vi "Display and Log Custom Device Error (Filtered).vi"(8 "error in (no error)":errorcluster, 9 "Note (empty)":string, 10 "Your code's public name":string) -> ()   [LabVIEW 2015, in "J1939 Addon Engine.lvlib" / "Error Handling API.lvlib"]
uses:
  Error Handling API.lvlib
  <vilib>/NI Veristand/Custom Device Tools/Custom Device Utility Library/NI VeriStand - Print Debug String.vi
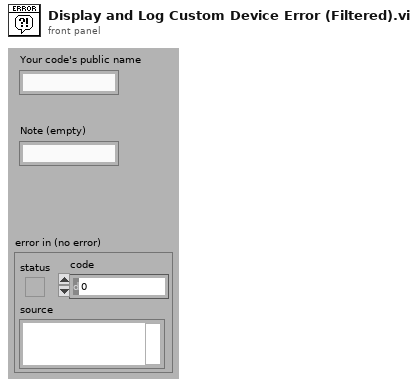
[diagram p1: front panel]
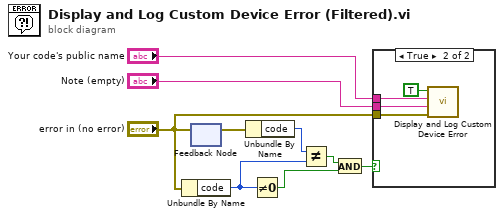
[diagram p0: block diagram]
diagram:
  n1 = Unbundle By Name("error in (no error)") -> ("code"=w8:i32)
  n2 = feedback #1() -> (w6:errorcluster)  [unwired: 1 in]
  n3 = feedback-in #1("error in (no error)") -> ()
  n4 = Unbundle By Name(w6) -> ("code"=w7:i32)
  n5 = Not Equal To 0?(x=w8) -> (x != 0?=w9:bool)
  n6 = Not Equal?(x=w7, y=w8) -> (x != y?=w4:bool)
  n7 = And(x=w4, y=w9) -> (x .and. y?=w5:bool)
  n8 = case shown="True" w5 {
    tunnel: "error in (no error)" -> [_ w13]
    tunnel: "Your code's public name" -> [_ w11]
    tunnel: "Note (empty)" -> [_ w10]
    frame False {
    }
    frame True {
      n9 = call "Display and Log Custom Device Error.vi"("error out"=w13, "Note (empty)"=w10, "Your code's public name"=w11, "Custom Device? (T)"=TRUE) -> ()  [unwired: 8 in]
    }
  }
